vi "myRIO_BRig_RT_comm_webdav_uploadFile__announce.vi"(6 "input_addText":bool, 8 "input_fileName_prefix":string, 10 "intput_fileName":string, 11 "intput_hSession":T1) -> (1 "output_Isuccess":bool, 3 "output_hSession":T1)   [LabVIEW 2014]
uses:
  <vilib>/WebDAVClient/Advanced/SessionHandle.ctl
  <vilib>/WebDAVClient/Advanced/Put File.vi
  <vilib>/WebDAVClient/NI_WebDAV.lvlib
panel:
  out "error out":errorcluster
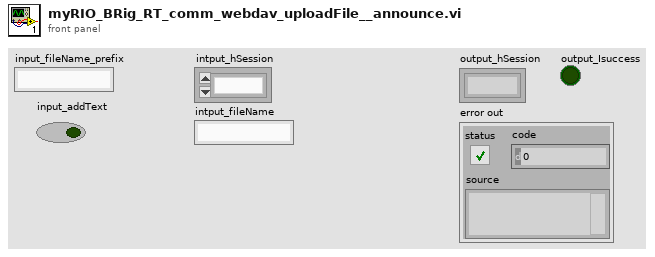
[diagram p1: front panel]
types:
  T1 = typedef "NI_WebDAV.lvlib/SessionHandle.ctl" = refnum<k1>
  T2 = enum16{"open", "replace", "create", "open or create", "replace or create", "replace or create with confirmation"}
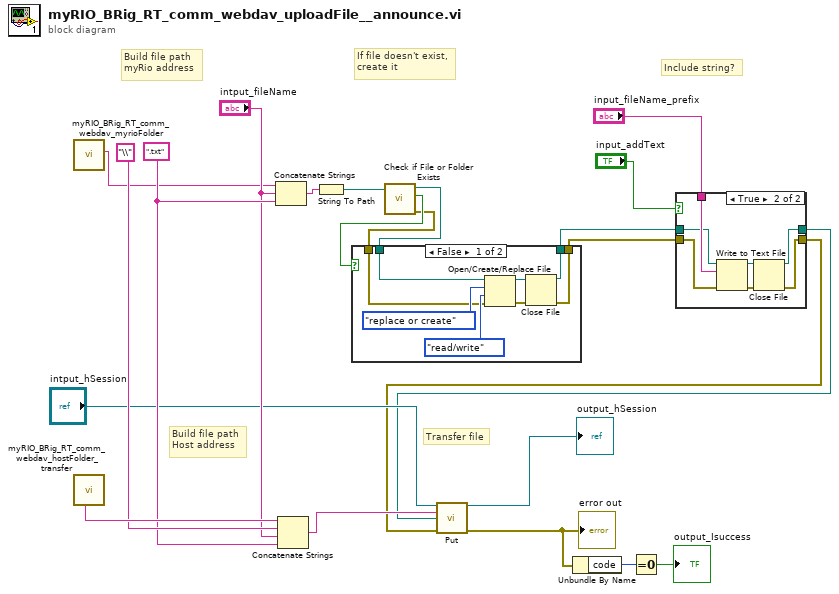
[diagram p0: block diagram]
diagram:
  w11 = ".txt" ("string")
  # "Transfer file"
  # "Build file path\nHost address"
  # "Include string?"
  # "If file doesn't exist,\ncreate it"
  # "Build file path\nmyRio address"
  n1 = call "myRIO_BRig_RT_comm_webdav_myrioFolder.vi"() -> ("output_myrioFolder"=w1:string)  [unwired: 11 in]
  n2 = call "myRIO_BRig_RT_comm_webdav_hostFolder_transfer.vi"() -> ("output_HostFolder"=w13:string)  [unwired: 11 in]
  n3 = Concatenate Strings(w1, "intput_fileName", w11) -> (w22:string)
  n4 = Concatenate Strings(w13, "\\" ("string"), "intput_fileName", w11) -> (w8:string)
  n5 = String To Path(string=w22) -> (path=w21:path)
  n6 = call <vilib>:"Check if File or Folder Exists.vi"("path"=w21) -> ("error out"=w18:errorcluster, "file or folder exists?"=w20:bool, "dup path"=w19:path)  [unwired: 8 in]
  n7 = case shown="False" w20 {
    tunnel: w19 -> [w28 w32]
    tunnel: w18 -> [w27 w31]
    tunnel: [w24 w32] -> w16
    tunnel: [w23 w31] -> w17
    frame False {
      n8 = Open/Create/Replace File(file path (use dialog)=w28, error in=w27, operation (0:open)=T2."replace or create", access (0:read/write)=enum16{"read/write", "read-only", "write-only"}."read/write") -> (refnum out=w25:refnum<file>, error out=w26:errorcluster)  [unwired: 2 in, 1 out]
      n9 = Close File(refnum=w25, error in=w26) -> (path=w24:path, error out=w23:errorcluster)
    }
    frame True {
    }
  }
  n10 = case shown="True" "input_addText" {
    tunnel: w17 -> [w33 w39]
    tunnel: w16 -> [w34 w40]
    tunnel: "input_fileName_prefix" -> [_ w41]
    tunnel: [w34 w36] -> w6
    tunnel: [w33 w35] -> w7
    frame False {
    }
    frame True {
      n11 = Write to Text File(file (use dialog)=w40, text=w41, error in=w39) -> (refnum out=w38:refnum<file>, error out=w37:errorcluster)  [unwired: 1 in, 1 out]
      n12 = Close File(refnum=w38, error in=w37) -> (path=w36:path, error out=w35:errorcluster)
    }
  }
  n13 = call-poly <vilib>:"Put.vi"("session handle"="intput_hSession", "relative uri"=w8, "local file path"=w6, "error in (no error)"=w7) -> ("session handle out"=→"output_hSession":T1, "error out"=w4:errorcluster)  [unwired: 9 in, 1 out]
  "error out" <- w4
  n14 = Unbundle By Name(w4) -> ("code"=w3:i32)
  n15 = Equal To 0?(x=w3) -> (x = 0?=→"output_Isuccess":bool)
